vi "X Scale Name Label Justification Read.vi"(4 "error in (no error)":errorcluster, 6 "Container State":T3, 7 "Display State In":T1) -> (0 "error out":errorcluster, 2 "Value":enum16{"Left", "Center", "Right"}(ring), 3 "Display State Out":T1)   [LabVIEW 2020, in "XY Plot Matrix.xctl"]
uses:
  <vilib>/Math Plots/2D Math Plots/XY Plot Matrix/XY Plot Matrix XCtrl/XY Plot Matrix.xctl
  <vilib>/_xctls/Container State.ctl
  <vilib>/Math Plots/2D Math Plots/XY Plot Matrix/XY Plot Matrix XCtrl/State.ctl
  <vilib>/Math Plots/2D Math Plots/XY Plot Matrix/XY Plot Matrix/XY Plot Matrix.lvclass
  e:/builds/penguin/labview/branches/2020/dev/dist/vi.lib/Math Plots/2D Math Plots/2D Plot/2D Plot/2D Plot.lvclass
  <vilib>/Math Plots/2D Math Plots/2D Plot/Action String/XYPlotMatrix Ctrl Act Queue.ctl
  <vilib>/Math Plots/2D Math Plots/2D Plot/Action String/XYPlotMatrix Ctrl Act Cluster.ctl
  <vilib>/Math Plots/2D Math Plots/2D Plot/Action String/2DMathPlot State Class.ctl
  <vilib>/Math Plots/2D Math Plots/2D Plot/2D Plot/2D Plot.lvclass
  <vilib>/_xctls/XControlSupport.lvlib
panel:
  # "Replace the Value Indicator below with an Indicator of desired type.\nDo not remove this Indicator or the others from the connector pane. \nDo not change the connector pane pattern.\nThe Value Indicator should always be the second terminal from top on the output side in the connector pane."
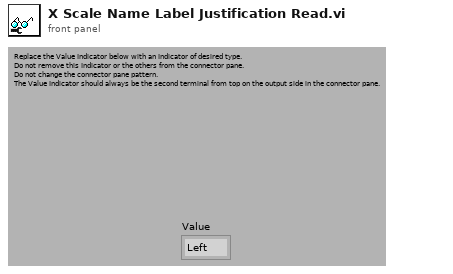
[diagram p1: front panel]
types:
  T1 = typedef "XY Plot Matrix.xctl/State.ctl" = cluster{"XY Plot Matrix.lvclass":refnum<class "XY Plot Matrix.lvclass">, "Control Ref Queue":T2, "Main Frame Color":u32}
  T2 = typedef "XYPlotMatrix Ctrl Act Queue.ctl" = refnum<queue>
  T3 = typedef "XControlSupport.lvlib/Container State.ctl" = cluster{"Indicator?":bool, "Run Mode?":bool, " Refnum":refnum<vi>}
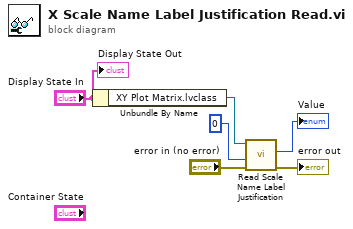
[diagram p0: block diagram]
diagram:
  n1 = Unbundle By Name("Display State In") -> ("XY Plot Matrix.lvclass"=w6:refnum<class "XY Plot Matrix.lvclass">)
  n2 = call <vilib>:"Read Scale Name Label Justification.vi"("error in (no error)"="error in (no error)", "Index"=0, "2D Plot.lvclass in"=w6) -> ("error out"=→"error out":errorcluster, "Name Label Justification"=→"Value":enum16{"Left", "Center", "Right"})  [unwired: 7 out]
  "Display State Out" <- "Display State In"
